vi "DSF.Memory.Cache.Plugin.Set Transfer Caches.vi"(8 "error in (no error)":errorcluster, 10 "Transfer Caches":refnum<class "DSF.Memory.Cache.Transfer.lvclass">[](array[class]), 11 "Plugin Cache in":refnum<class "DSF.Memory.Cache.Plugin.lvclass">) -> (0 "error out":errorcluster, 3 "Plugin Cache out":refnum<class "DSF.Memory.Cache.Plugin.lvclass">)   [LabVIEW 2016, in "DSF.Memory.lvlib" / "DSF.Memory.Cache.Plugin.lvclass"]
uses:
  DSF.Memory.Cache.Plugin.lvclass
  DSF.Memory.Cache.Transfer.lvclass
  DSF.Memory.Cache.Plugin.lvclass/DSF.Memory.Cache.Plugin.ctl
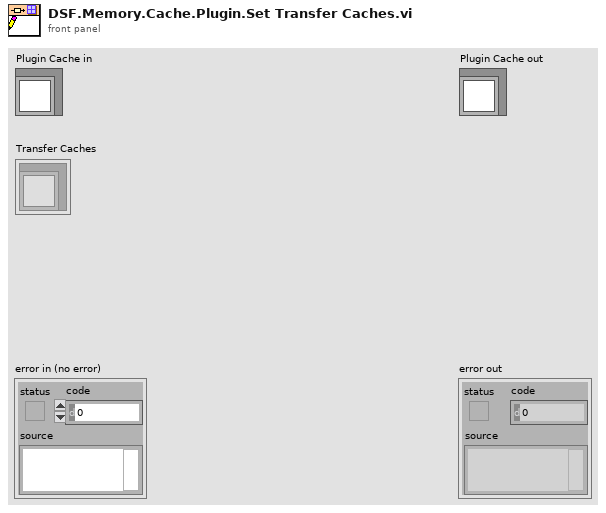
[diagram p1: front panel]
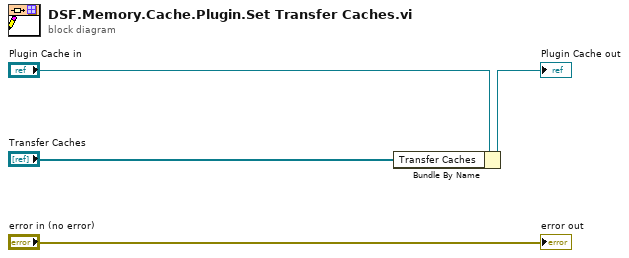
[diagram p0: block diagram]
diagram:
  n1 = Bundle By Name(cluster="Plugin Cache in", "Transfer Caches"="Transfer Caches") -> (→"Plugin Cache out":refnum<class "DSF.Memory.Cache.Plugin.lvclass">)
  "error out" <- "error in (no error)"
